vi "Parse Data Channels.vi"(8 "error in":errorcluster, 10 "DataChan Type":T1, 11 "Device Reference in":T5 format="%.0x") -> (0 "error out":errorcluster, 2 "Channels":T2 {"BD Refs"."Data Reference" format="%.0x"}, 3 "Device Reference out":T5 format="%.0x")   [LabVIEW 2017, in "RefMem DMA Custom Device.lvlib"]
uses:
  <vilib>/NI Veristand/Custom Device API/Custom Device Item Ref.ctl
  Shared/RT Chan Cluster.ctl
  <vilib>/NI Veristand/Custom Device API/Block Data Reference.ctl
  <vilib>/NI Veristand/Custom Device API/Data Reference.ctl
  Shared/Data Channel Type.ctl
  <vilib>/NI Veristand/Custom Device API/Data Access Type.ctl
  <vilib>/NI Veristand/Custom Device API/Get Item Property (U32).vi
  <vilib>/NI Veristand/Custom Device Tools/Custom Device Utility Library/NI VeriStand - Search for All Items by Property.vi
  Shared/Global.vi
  RefMem DMA Custom Device.lvlib
  <vilib>/NI VeriStand/Custom Device Tools/Custom Device Utility Library/Custom Device Utility Library.lvlib
  Shared/GE_RM_Shared.lvlib
  <vilib>/NI Veristand/Custom Device API/Custom Device API.lvlib
  System Explorer/GE_RM_System Explorer.lvlib
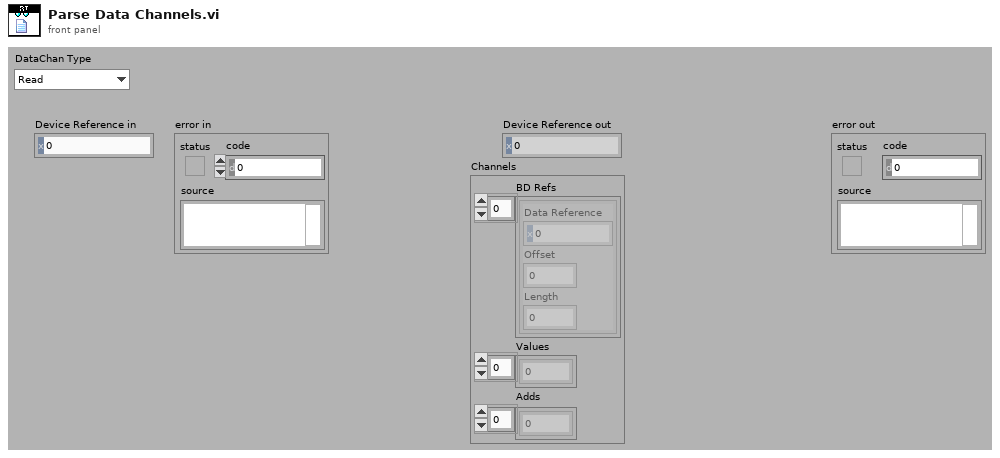
[diagram p1: front panel]
types:
  T1 = typedef "GE_RM_System Explorer.lvlib/Data Channel Type.ctl" = enum16{"Read", "Write"}
  T2 = typedef "GE_RM_Shared.lvlib/RT Chan Cluster.ctl" = cluster{"BD Refs":T3[], "Values":dbl[], "Adds":u32[]}
  T3 = typedef "Custom Device API.lvlib/Block Data Reference.ctl" = cluster{"Data Reference":T4, "Offset":u64, "Length":u64}
  T4 = typedef "Custom Device API.lvlib/Data Reference.ctl" = i32
  T5 = typedef "Custom Device API.lvlib/Custom Device Item Ref.ctl" = u64
  T6 = typedef "Custom Device API.lvlib/Data Access Type.ctl" = enum16{"Read", "Write"}
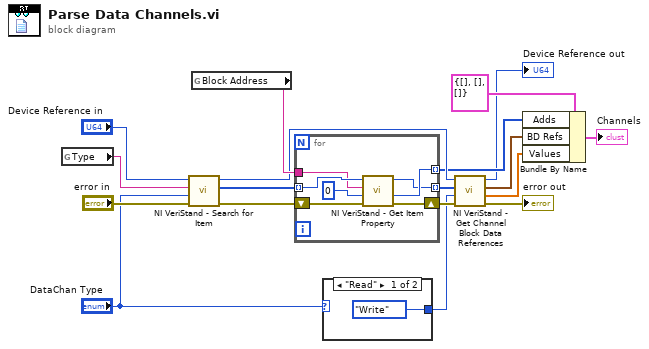
[diagram p0: block diagram]
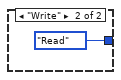
[diagram p2: hidden frame]
diagram:
  n1 = global read "Global.vi" "Type"() -> (w3:string)
  n2 = call-poly <vilib>:"NI VeriStand - Search for Item.vi"("error in"="error in", "Property Value"="DataChan Type", "Property Name"=w3, "Section Ref in"="Device Reference in") -> ("error out"=w15:errorcluster, "Item Refs"=w16:T5[], "Section Ref out"=w13:T5)  [unwired: 4 in, 1 out]
  n3 = global read "Global.vi" "Block Address"() -> (w17:string)
  n4 = for {
    shift-right: [w20] -> w12
    shift-left: w15 -> [w25]
    tunnel: w16 -> [w24] mode=indexing
    tunnel: w17 -> [w23]
    tunnel: [w21] -> w5 mode=indexing
    tunnel: [w19] -> w11 mode=indexing
    n5 = call-poly <vilib>:"NI VeriStand - Get Item Property.vi"("error in (no error)"=w25, "Default Value"=u32 0, "Property Name"=w23, "Item Ref in"=w24) -> ("error out"=w20:errorcluster, "Value"=w21:u32, "Item Ref out"=w19:T5)  [unwired: 4 in, 1 out]
  }
  n6 = case shown="\"Read\"" "DataChan Type" {
    tunnel: [Data_Access_Type."Write" ("Access") Data_Access_Type."Read" ("Access")] -> w10
    frame "Read" {
    }
    frame "Write" {
    }
  }
  n7 = call <vilib>:"NI VeriStand - Get Channel Block Data References.vi"("error in (no error)"=w12, "Access"=w10, "Channel Refs"=w11, "Device Ref in"=w13) -> ("error out"=→"error out":errorcluster, "Values Array"=w7:dbl[], "Block Data Refs"=w8:T3[], "Device Ref out"=→"Device Reference out":T5)  [unwired: 4 in]
  n8 = Bundle By Name(cluster=T2 {"BD Refs"=[], "Values"=[], "Adds"=[]} ("Read Chns"), "Adds"=w5, "BD Refs"=w8, "Values"=w7) -> (→"Channels":T2)
